vi "SVPO Peak Level (1 Ch DBL WDT).vi"(6 "restart averaging? (F)":bool, 11 "scaled signal [EU]":waveform(dbl)={"t0"=timestamp(0 s since 1904-01-01), "dt"=0.0, "Y"=[]}) -> (1 "minimum level [EU]":dbl=nan, 2 "maximum level [EU]":dbl=nan, 3 "peak level [EU]":dbl=nan, 4 "duration [s]":dbl, 5 "timestamp":timestamp)   [LabVIEW 2017, in "SoundVib_VibrationLevel.lvlib"]
doc: "Uses a peak detector and computes the level of scaled time waveform signals and scaled array signals. <B>scaled signal [EU]</B> should have a zero DC component. You can attenuate the DC component with hardware AC-coupling filters and with software high-pass filters. Use this VI on embedded targets that have limited computational resources. Wire data to the scaled signal [EU] input to determine the polymorphic instance to use or manually select the instance."
uses:
  <vilib>/addons/Sound and Vibration/svt_Level/SoundVib_VibrationLevel.lvlib
  <vilib>/addons/Sound and Vibration/svt_Level/SVPO Peak Level (1 Ch DBL Array) with IC.vi
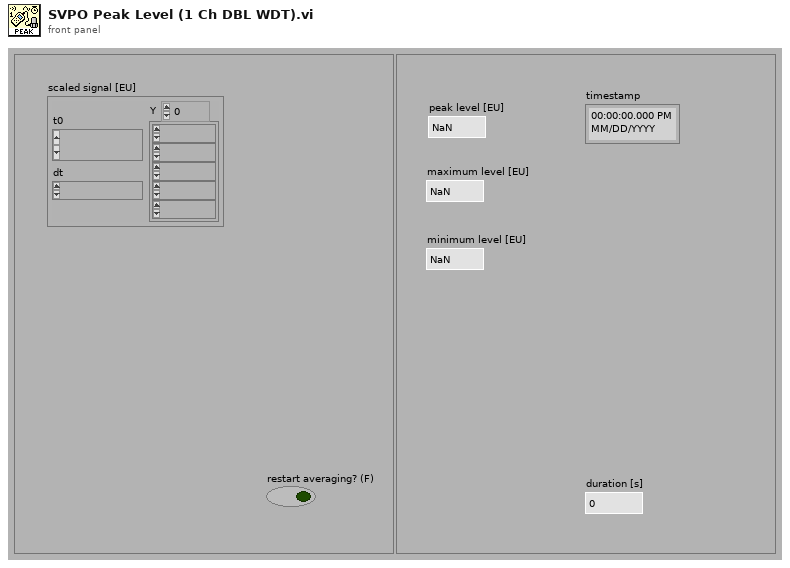
[diagram p1: front panel]
types:
  T1 = typedef "svc_Peak Level State.ctl" = cluster{"historical max":dbl, "historical min":dbl, "cumulative size":u64, "timestamp":timestamp}
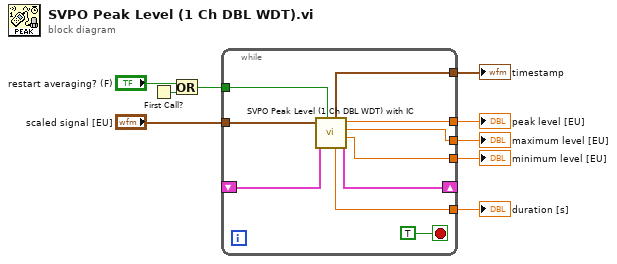
[diagram p0: block diagram]
diagram:
  n1 = First Call?() -> (First Call?: T/F=w8:bool)
  n2 = Or(x="restart averaging? (F)", y=w8) -> (x .or. y?=w5:bool)
  n3 = while {
    tunnel: "scaled signal [EU]" -> [w17]
    tunnel: [w13] -> w6
    tunnel: w5 -> [w16]
    tunnel: [w18] -> w4
    shift-right: [w14] -> _
    shift-left: _ -> [w15]
    tunnel: [w12] -> w3
    tunnel: [w11] -> w2
    tunnel: [w10] -> w1
    stop <- TRUE stop-if-true
    n4 = call <vilib>:"SVPO Peak Level (1 Ch DBL WDT) with IC.vi"("restart averaging? (F)"=w16, "initial conditions"=w15, "scaled signal [EU]"=w17) -> ("final conditions"=w14:T1, "minimum level [EU]"=w10:dbl, "maximum level [EU]"=w11:dbl, "peak level [EU]"=w12:dbl, "duration [s]"=w13:dbl, "timestamp"=w18:timestamp)  [unwired: 3 in]
  }
  "timestamp" <- w4
  "duration [s]" <- w6
  "peak level [EU]" <- w3
  "minimum level [EU]" <- w1
  "maximum level [EU]" <- w2
